vi "Check for Names v2.vi"(0 "New Name":string, 1 "Name List":string[](array[string]), 2 "Empty Plots?":bool[](array[boolean]), 3 "Error In":errorcluster) -> (5 "New Name List":string[](array[string]), 6 "New Name":string, 7 "Checked Array":bool[](array[boolean]), 9 "Error Out":errorcluster)   [LabVIEW 2019]
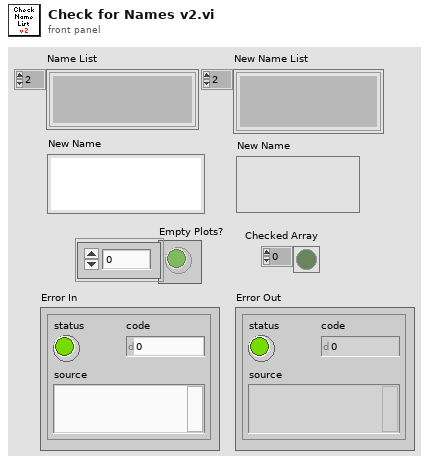
[diagram p1: front panel]
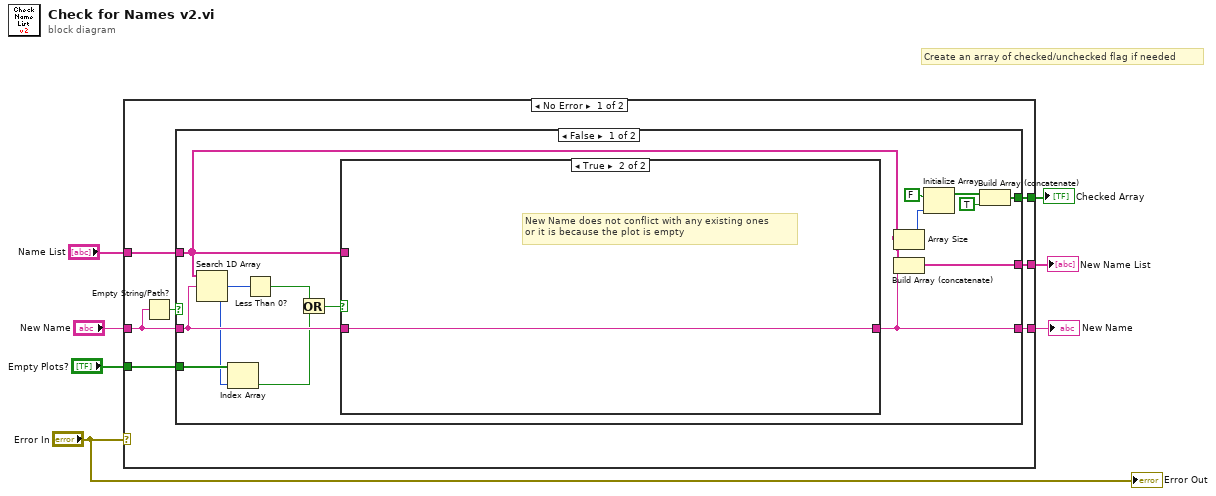
[diagram p0: block diagram]
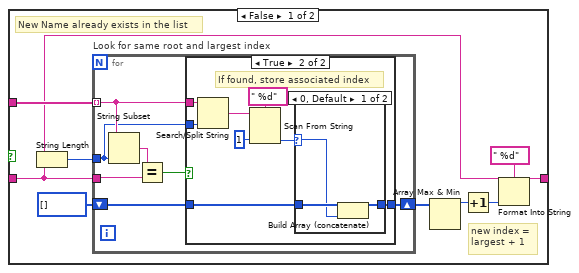
[diagram p2: hidden frame]
diagram:
  # "Create an array of checked/unchecked flag if needed"
  n1 = case shown="No Error" "Error In" {
    tunnel: [w14 w61] -> w7
    tunnel: [w13 w62] -> w6
    tunnel: [w12 _] -> w5
    tunnel: "Name List" -> [w11 w62]
    tunnel: "New Name" -> [w10 w61]
    tunnel: "Empty Plots?" -> [w8 _]
    frame No Error {
      n2 = Empty String/Path?(string/path=w10) -> (empty?=w9:bool)
      n3 = case shown="False" w9 {
        tunnel: [w28 w59] -> w14
        tunnel: [w27 w60] -> w13
        tunnel: [w22 _] -> w12
        tunnel: w11 -> [w21 w60]
        tunnel: w10 -> [w20 w59]
        tunnel: w8 -> [w19 _]
        frame False {
          n4 = Search 1D Array(1D array=w21, element=w20) -> (index of element=w18:i32)  [unwired: 1 in]
          n5 = Index Array(array=w19, index=w18) -> (element=w16:bool)
          n6 = Less Than 0?(x=w18) -> (x < 0?=w17:bool)
          n7 = Or(x=w17, y=w16) -> (x .or. y?=w15:bool)
          n8 = case shown="True" w15 {
            tunnel: w20 -> [w29 w58]
            tunnel: [w32 w58] -> w28
            tunnel: w21 -> [w37 _]
            frame False {
              # "new index =\nlargest + 1"
              # "New Name already exists in the list"
              n9 = String Length(string=w29) -> (length=w31:i32)
              n10 = for "Look for same root and largest index" {
                tunnel: w37 -> [w39] mode=indexing
                tunnel: w29 -> [w41]
                shift-right: [w43] -> w35
                shift-left: i32[] [] -> [w44]
                tunnel: w31 -> [w38]
                n11 = String Subset(string=w39, length (rest)=w38) -> (substring=w42:string)  [unwired: 1 in]
                n12 = Equal?(x=w42, y=w41) -> (x = y?=w40:bool)
                n13 = case shown="True" w40 {
                  tunnel: w44 -> [w45 w52]
                  tunnel: [w45 w51] -> w43
                  tunnel: w39 -> [_ w50]
                  tunnel: w38 -> [_ w49]
                  frame False {
                  }
                  frame True {
                    # "If found, store associated index"
                    n14 = Search/Split String(string=w50, offset (0)=w49) -> (match + rest of string=w48:string)  [unwired: 1 in, 2 out]
                    n15 = Scan From String(format string=" %d" ("Format String"), input string=w48, default 1=1 ("Default Value 1")) -> (output 1=w46:i32)  [unwired: 2 in, 3 out]
                    n16 = case shown="0, Default" w46 {
                      selector: w46 -> [w54 _]
                      tunnel: w52 -> [w56 w57]
                      tunnel: [w55 w57] -> w51
                      frame 0, Default {
                        n17 = Build Array (concatenate)(w56, w54) -> (w55:i32[])
                      }
                      frame -1 {
                        # "not an index"
                      }
                    }
                  }
                }
              }
              n18 = Array Max & Min(array=w35) -> (max value=w34:i32)  [unwired: 3 out]
              n19 = Increment(x=w34) -> (x+1=w33:i32)
              n20 = Format Into String(format string=" %d" ("Format String"), initial string=w29, w33) -> (resulting string=w32:string)  [unwired: 1 in, 1 out]
            }
            frame True {
              # "New Name does not conflict with any existing ones\nor it is because the plot is empty"
            }
          }
          n21 = Array Size(array=w21) -> (size(s)=w26:i32)
          n22 = Build Array (concatenate)(w21, w28) -> (w27:string[])
          n23 = Initialize Array(FALSE, w26) -> (w24:bool[])
          n24 = Build Array (concatenate)(w24, TRUE ("Input Element")) -> (w22:bool[])
        }
        frame True {
        }
      }
    }
    frame Error {
    }
  }
  "New Name" <- w7
  "New Name List" <- w6
  "Checked Array" <- w5
  "Error Out" <- "Error In"
